vi "Generate Trajectory for Alignment.vi"(8 "Setpoints":T2={"x setpoint"=0.559167, "y setpoint"=0.559167, "th setpoint"=0.559167}, 9 "th":dbl=-1.4450115280878395, 10 "y":dbl=-0.7874329977815421, 11 "x":dbl=-0.0038485573430510045) -> (3 "Trajectory Data Out":T4(array[cluster])=[{"Segment Name"="Linear 0", "Type"=enum."Accel Straight", "Traj Pos Points"=[{"x"=-0.012626500873375458, "y"=-2.5834416764415944, "th"=-1.4450114965438843}, {"x"=-0.0066265008733754575, "y"=-2.5834416764415944, "th"=-1.3656081390380859}, {"x"=0.005373499126624543, "y"=-2.5834416764415944, "th"=-1.2862047815322877}, {"x"=0.023373499126624543, "y"=-2.5834416764415944, "th"=-1.2068014240264893}, {"x"=0.047373499126624544, "y"=-2.5834416764415944, "th"=-1.1273980665206909}, {"x"=0.07737349912662454, "y"=-2.5834416764415944, "th"=-1.0479947090148927}, {"x"=0.11337349912662455, "y"=-2.5834416764415944, "th"=-0.9685913515090943}, {"x"=0.14937349912662456, "y"=-2.5834416764415944, "th"=-0.8891879940032958}, {"x"=0.18537349912662457, "y"=-2.5834416764415944, "th"=-0.8097846364974975}, {"x"=0.22137349912662457, "y"=-2.5834416764415944, "th"=-0.7303812789916992}, {"x"=0.25737349912662455, "y"=-2.5834416764415944, "th"=-0.650977921485901}, {"x"=0.2933734991266246, "y"=-2.5834416764415944, "th"=-0.5715745639801026}, {"x"=0.3293734991266246, "y"=-2.5834416764415944, "th"=-0.49217120647430435}, {"x"=0.36537349912662465, "y"=-2.5834416764415944, "th"=-0.41276784896850605}, {"x"=0.4013734991266247, "y"=-2.5834416764415944, "th"=-0.33336449146270763}, {"x"=0.4373734991266247, "y"=-2.5834416764415944, "th"=-0.2539611339569092}, {"x"=0.46737349912662474, "y"=-2.5834416764415944, "th"=-0.1745577764511108}, {"x"=0.49137349912662476, "y"=-2.5834416764415944, "th"=-0.0951544189453124}, {"x"=0.5093734991266248, "y"=-2.5834416764415944, "th"=-0.01575106143951399}, {"x"=0.5213734991266248, "y"=-2.5834416764415944, "th"=-0.01575106143951399}, {"x"=0.5273734991266248, "y"=-2.5834416764415944, "th"=0.0}], "Traj Vel Points"=[{"V"=0.3, "Omega"=0.0, "V vector"={"y"=-0.0075652604517563735, "x"=0.2999045962206933}}, {"V"=0.6, "Omega"=3.970167875289917, "V vector"={"y"=-0.014299261055195281, "x"=0.599829585076691}}, {"V"=0.8999999999999999, "Omega"=3.970167875289917, "V vector"={"y"=-0.02020196061600483, "x"=0.8997732385369489}}, {"V"=1.2, "Omega"=3.970167875289917, "V vector"={"y"=-0.02527332113298065, "x"=1.1997338284965167}}, {"V"=1.5, "Omega"=3.970167875289917, "V vector"={"y"=-0.029513307798150146, "x"=1.4997096267820686}}, {"V"=1.8, "Omega"=3.970167875289917, "V vector"={"y"=-0.03292188899688745, "x"=1.7996989051574368}}, {"V"=1.8, "Omega"=3.970167875289917, "V vector"={"y"=-0.0304277454068736, "x"=1.799742801710693}}, {"V"=1.8, "Omega"=3.970167875289917, "V vector"={"y"=-0.0279335433779409, "x"=1.7997832417139439}}, {"V"=1.8, "Omega"=3.970167875289917, "V vector"={"y"=-0.025439287700403847, "x"=1.7998202250895217}}, {"V"=1.8, "Omega"=3.970167875289917, "V vector"={"y"=-0.022944983164679984, "x"=1.7998537517663964}}, {"V"=1.8, "Omega"=3.970167875289917, "V vector"={"y"=-0.020450634561280663, "x"=1.7998838216801776}}, {"V"=1.8, "Omega"=3.970167875289917, "V vector"={"y"=-0.017956246680801907, "x"=1.7999104347731136}}, {"V"=1.8, "Omega"=3.970167875289917, "V vector"={"y"=-0.01546182431391515, "x"=1.7999335909940917}}, {"V"=1.8, "Omega"=3.970167875289917, "V vector"={"y"=-0.012967372251358066, "x"=1.7999532902986384}}, {"V"=1.8, "Omega"=3.970167875289917, "V vector"={"y"=-0.010472895283925358, "x"=1.7999695326489202}}, {"V"=1.5, "Omega"=3.970167875289917, "V vector"={"y"=-0.0066486651687163115, "x"=1.4999852650114516}}, {"V"=1.2, "Omega"=3.970167875289917, "V vector"={"y"=-0.00365592386522792, "x"=1.1999944309123654}}, {"V"=0.8999999999999999, "Omega"=3.970167875289917, "V vector"={"y"=-0.0014946814304914382, "x"=0.8999987588477115}}, {"V"=0.5999999999999999, "Omega"=3.970167875289917, "V vector"={"y"=-0.00016494472760446378, "x"=0.5999999773276968}}, {"V"=0.2999999999999999, "Omega"=0.0, "V vector"={"y"=-8.247236380223188e-05, "x"=0.29999998866384836}}, {"V"=0.0, "Omega"=0.0, "V vector"={"y"=0.0, "x"=0.0}}], "Accel Index"=7, "Decel Index"=15}, {"Segment Name"="", "Type"=enum."Accel Straight", "Traj Pos Points"=[], "Traj Vel Points"=[], "Accel Index"=0, "Decel Index"=0}])   [LabVIEW 2023]
uses:
  bordeaux-pathinator/Bordeaux/Types/Segment Type.ctl
  bordeaux-pathinator/Bordeaux/Types/Limits.ctl
  bordeaux-pathinator/Bordeaux/Types/Angluar Limits.ctl
  bordeaux-pathinator/Bordeaux/Types/Drive Type.ctl
panel:
  in  "Limits":T1={"Velocity (fps)"=6.0, "Accel (fps^2)"=30.0, "Jerk (fps^3)"=4000.0, "StoopidFast (fps)"=6.0} {"StoopidFast (fps)" min=0.0; "Jerk (fps^3)" min=0.0 step=1.0; "Accel (fps^2)" min=0.0; "Velocity (fps)" min=0.0}
  in  "y 2":dbl=2.25 format="%#_13g"
  out "Error":cluster{dbl, dbl, "th":dbl}
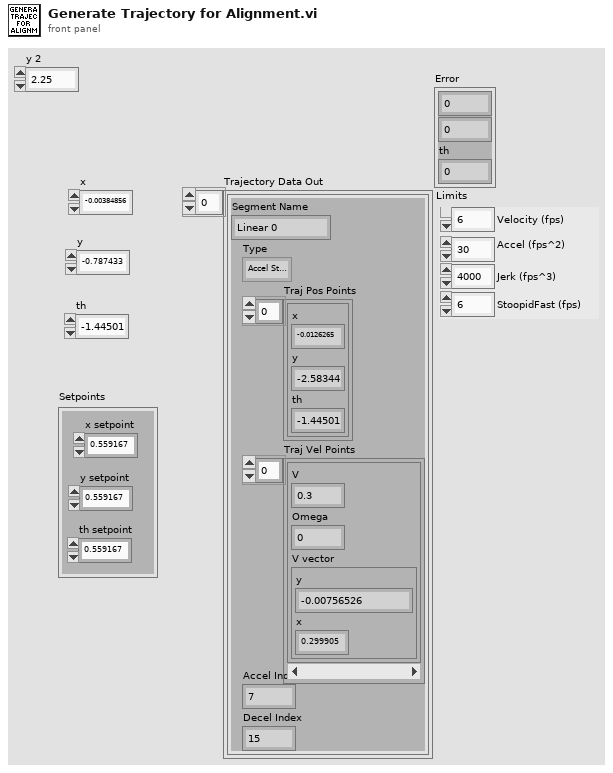
[diagram p1: front panel]
types:
  T1 = typedef "Limits.ctl" = cluster{"Velocity (fps)":dbl, "Accel (fps^2)":dbl, "Jerk (fps^3)":dbl, "StoopidFast (fps)":dbl}
  T2 = cluster{"x setpoint":dbl, "y setpoint":dbl, "th setpoint":dbl}
  T3 = typedef "Segment Type.ctl" = enum16{"Accel Straight", "Const Straight", "Blend", "Circle", "Bezier"}
  T4 = cluster{"Segment Name":string, "Type":T3, "Traj Pos Points":cluster{"x":dbl, "y":dbl, "th":dbl}[], "Traj Vel Points":cluster{"V":dbl, "Omega":dbl, "V vector":cluster{"y":dbl, "x":dbl}}[], "Accel Index":i32, "Decel Index":i32}[]
  T5 = cluster{"vInitial (fps)":dbl, "vFinal (fps)":dbl}
  T6 = typedef "Drive Type.ctl" = enum16{"Nonholonomic", "Holonomic"}
  T7 = typedef "Angluar Limits.ctl" = cluster{"Velocity (deg/s)":dbl, "Accel (deg/s^2)":dbl, "Jerk (deg/s^3)":dbl}
  T8 = cluster{"x setpoint":dbl, "y setpoint":dbl, "th setpoint":dbl}[]
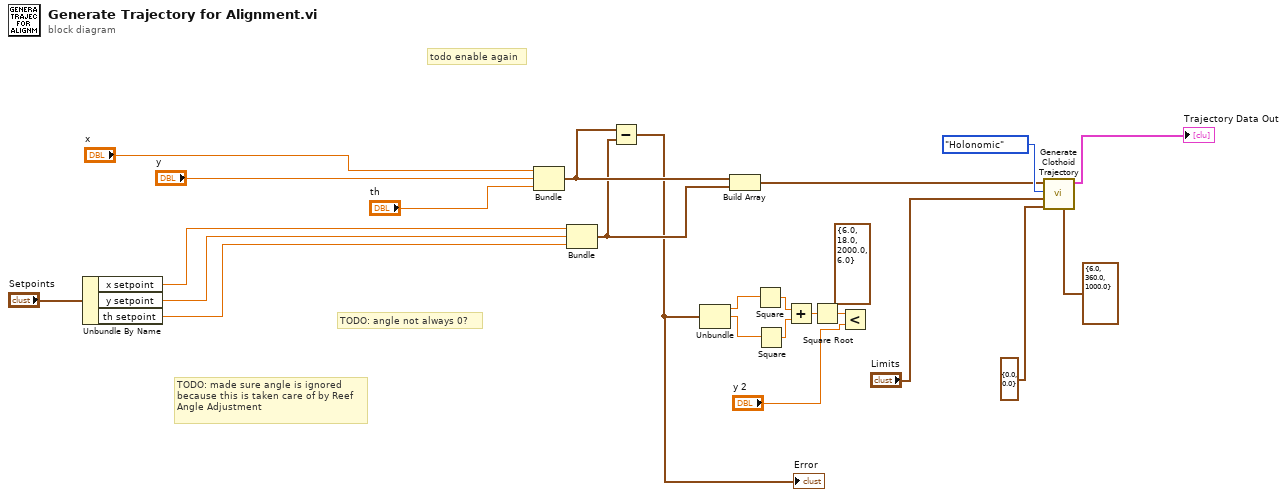
[diagram p0: block diagram]
diagram:
  (unwired) T1 {"Velocity (fps)"=6.0, "Accel (fps^2)"=18.0, "Jerk (fps^3)"=2000.0, "StoopidFast (fps)"=6.0} ("Limits")
  # "TODO: made sure angle is ignored\nbecause this is taken care of by Reef\nAngle Adjustment"
  # "todo enable again"
  # "TODO: angle not always 0?"
  n1 = Unbundle By Name("Setpoints") -> ("x setpoint"=w18:dbl, "y setpoint"=w17:dbl, "th setpoint"=w5:dbl)
  n2 = Bundle("x"="x", "y"="y", "th"="th") -> (w15:cluster{"x":dbl, "y":dbl, "th":dbl})  [unwired: 1 in]
  n3 = Bundle("x setpoint"=w18, "y setpoint"=w17, "th setpoint"=w5) -> (w14:T2)  [unwired: 1 in]
  n4 = Subtract(x=w15, y=w14) -> (x-y=w13:cluster{dbl, dbl, dbl})
  "Error" <- w13
  n5 = Unbundle(w13) -> (w12:dbl, w11:dbl)  [unwired: 1 out]
  n6 = Build Array(w15, w14) -> (w16:T8)
  n7 = Square(x=w12) -> (x^2=w9:dbl)
  n8 = Square(x=w11) -> (x^2=w8:dbl)
  n9 = Add(x=w9, y=w8) -> (x+y=w10:dbl)
  n10 = Square Root(x=w10) -> (sqrt(x)=w7:dbl)
  n11 = Less?(x=w7, y="y 2") -> ()  [unwired: 1 out]
  n12 = call "Generate Clothoid Trajectory.vi"("Angular Limits"=T7 {"Velocity (deg/s)"=6.0, "Accel (deg/s^2)"=360.0, "Jerk (deg/s^3)"=1000.0}, "Drive Type"=Drive_Type."Holonomic", "Conditions"=T5 {"vInitial (fps)"=0.0, "vFinal (fps)"=0.0}, "Limits"="Limits", "WayPoints"=w16) -> ("Trajectory Data Out"=→"Trajectory Data Out":T4)  [unwired: 3 in, 3 out]
